vi "TCP Client2 一对多通讯.vi"() -> ()   [LabVIEW 2015]
panel:
  in  "端口":u16
  in  "address":string
  out "Client 2":dbl[](graph)
  in  "stop":bool
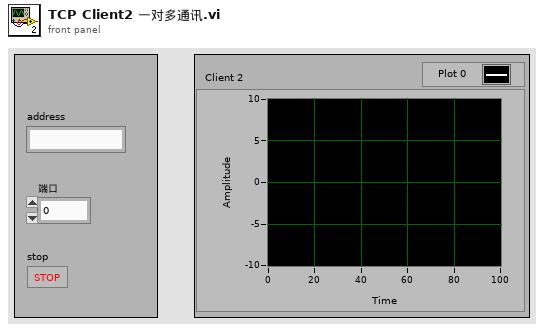
[diagram p1: front panel]
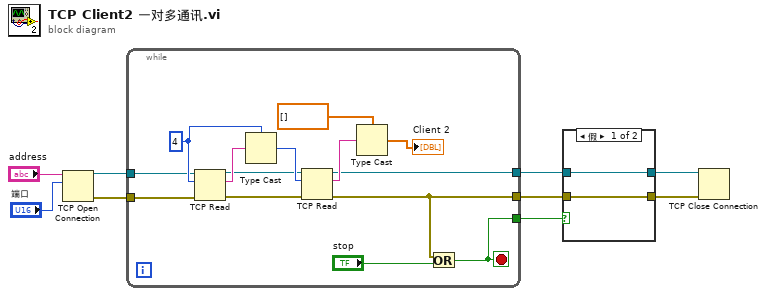
[diagram p0: block diagram]
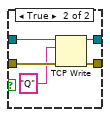
[diagram p2: hidden frame]
diagram:
  n1 = TCP Open Connection(address="address", remote port or service name="端口") -> (connection ID=w9:refnum<k5>, error out=w8:errorcluster)  [unwired: 3 in]
  n2 = while {
    tunnel: w9 -> [w15]
    tunnel: w8 -> [w14]
    tunnel: [w10] -> w5
    tunnel: [w13] -> w4
    tunnel: [w12] -> w3
    stop <- w12 stop-if-true
    w23 = 4
    n3 = TCP Read(connection ID=w15, bytes to read=w23, error in (no error)=w14) -> (connection ID out=w17:refnum<k5>, data out=w22:string, error out=w16:errorcluster)  [unwired: 2 in]
    n4 = Type Cast(type=w23, x=w22) -> (*(type *) &x=w21:i32)
    n5 = TCP Read(connection ID=w17, bytes to read=w21, error in (no error)=w16) -> (connection ID out=w13:refnum<k5>, data out=w20:string, error out=w10:errorcluster)  [unwired: 2 in]
    n6 = Type Cast(type=dbl[] [], x=w20) -> (*(type *) &x=→"Client 2":dbl[])
    n7 = Or(x=w10, y="stop") -> (x .or. y?=w12:bool)
  }
  n8 = case shown="假" w3 {
    tunnel: w5 -> [w24 w30]
    tunnel: w4 -> [w25 w29]
    tunnel: [w25 w28] -> w2
    tunnel: [w24 w27] -> w1
    frame False {
    }
    frame True {
      n9 = TCP Write(connection ID=w29, data in="Q", error in (no error)=w30) -> (connection ID out=w28:refnum<k5>, error out=w27:errorcluster)  [unwired: 1 in, 1 out]
    }
  }
  n10 = TCP Close Connection(connection ID=w2, error in (no error)=w1) -> ()  [unwired: 1 in, 2 out]
